vi "programa 2 Proto.vi"() -> ()   [LabVIEW 2011]
panel:
  in  "stop":bool
  out "ledn 3":bool
  out "ledn 2":bool
  out "ledn 1":bool
  in  "led 3":bool
  in  "led 2":bool
  in  "led 1":bool
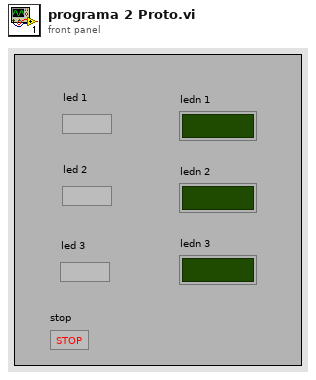
[diagram p1: front panel]
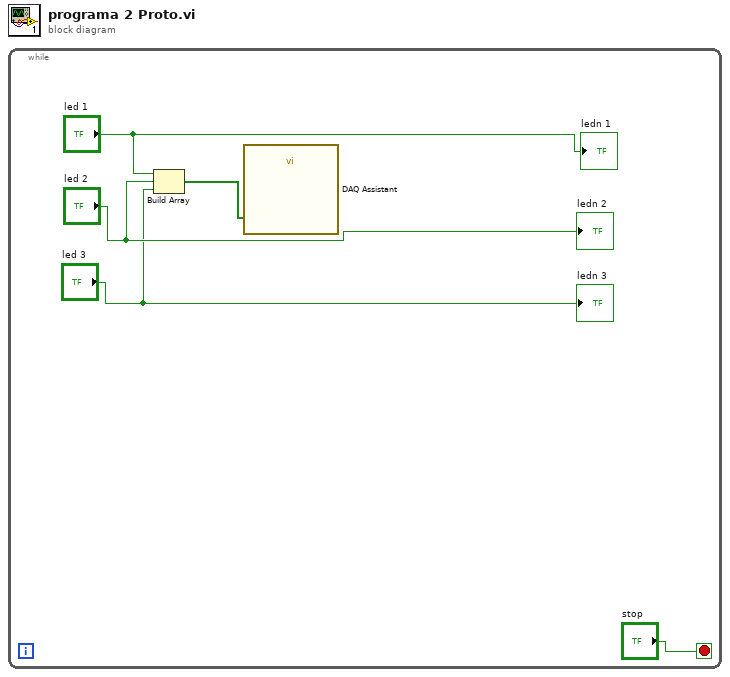
[diagram p0: block diagram]
diagram:
  n1 = while {
    stop <- "stop" stop-if-true
    n2 = Build Array("led 1", "led 2", "led 3") -> (w1:bool[])
    n3 = call "DAQ Assistant"("data"=w1) -> ()  [unwired: 17 in, 2 out]
    "ledn 1" <- "led 1"
    "ledn 2" <- "led 2"
    "ledn 3" <- "led 3"
  }
